vi "StrToNum.vi"(1 "String":string) -> (0 "number":dbl)   [LabVIEW 2018]
doc: "Zamienia string z E w liczbê."
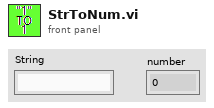
[diagram p1: front panel]
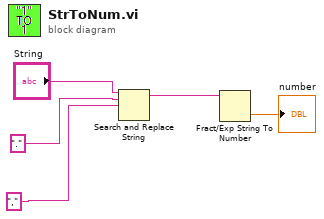
[diagram p0: block diagram]
diagram:
  n1 = Search and Replace String(input string="String", search string=".", replace string=",") -> (result string=w2:string)  [unwired: 5 in, 3 out]
  n2 = Fract/Exp String To Number(string=w2) -> (number=→"number":dbl)  [unwired: 3 in, 1 out]
